vi "Hindbrain.vi"() -> ()   [LabVIEW 2012]
panel:
  in  "VISA resource name":refnum<visa-resource-name>="COM6"
  in  "PC Status":i32=1
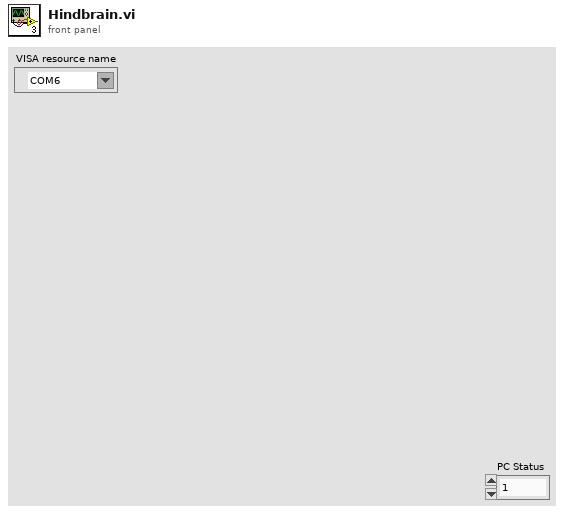
[diagram p1: front panel]
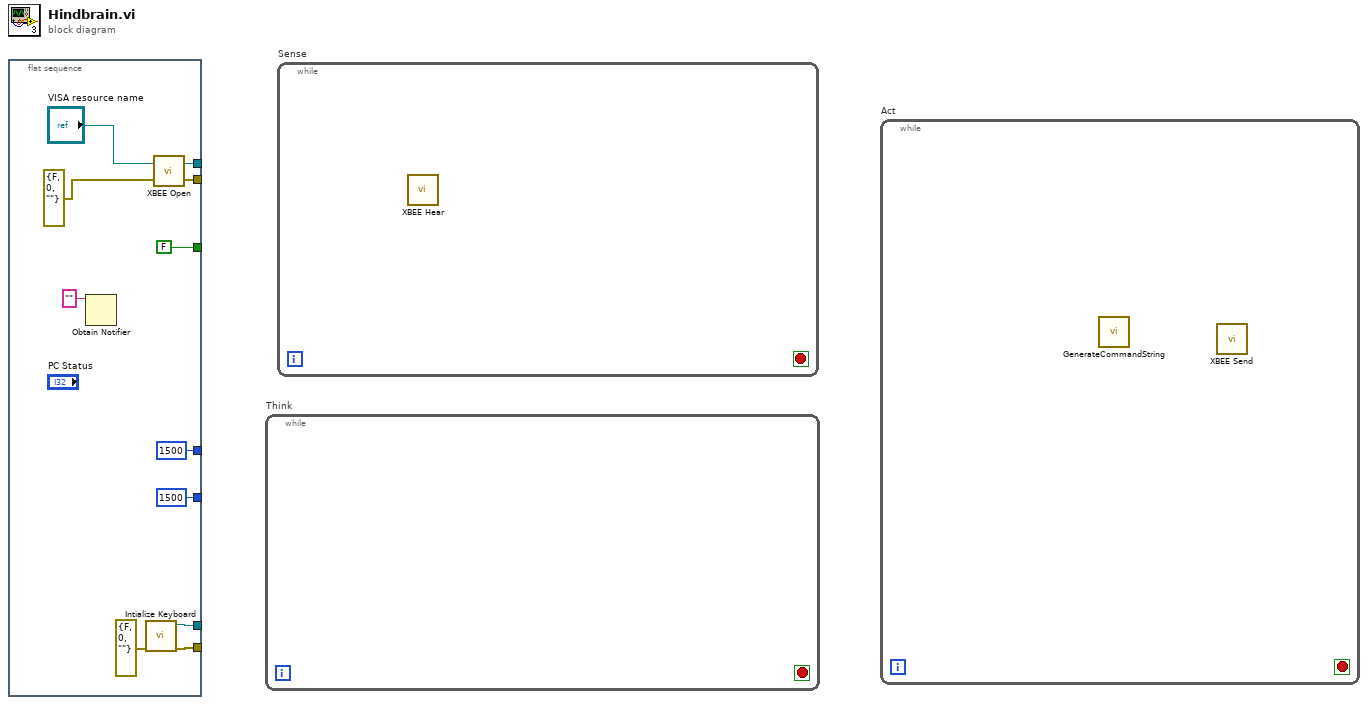
[diagram p0: block diagram]
diagram:
  n1 = flat-sequence {
    tunnel: [w11] -> _
    tunnel: [w10] -> _
    tunnel: [FALSE] -> _
    tunnel: [w8] -> _
    tunnel: [w6] -> _
    tunnel: [1500] -> _
    tunnel: [1500] -> _
    frame #0 {
      n2 = Obtain Notifier(name (unnamed)="") -> ()  [unwired: 3 in, 3 out]
      n3 = call <vilib>:"Intialize Keyboard.vi"("error in (no error)"=errorcluster {"status"=FALSE, "code"=0, "source"=""}) -> ("error out"=w8:errorcluster, "device ID"=w6:refnum<k1>)  [unwired: 9 in]
      n4 = call "XBEE Open.vi"("error in"=errorcluster {"status"=FALSE, "code"=0, "source"=""}, "VISA resource name"="VISA resource name") -> ("error out"=w10:errorcluster, "VISA resource name out"=w11:refnum<visa-resource-name>)
    }
  }
  n5 = while "Think" {
    stop <- _ stop-if-true
  }
  n6 = while "Sense" {
    stop <- _ stop-if-true
    n7 = call "XBEE Hear.vi"() -> ()  [unwired: 2 in, 4 out]
  }
  n8 = while "Act" {
    stop <- _ stop-if-true
    n9 = call "GenerateCommandString.vi"() -> ()  [unwired: 12 in]
    n10 = call "XBEE Send.vi"() -> ()  [unwired: 3 in, 3 out]
  }
